vi "Grenzen und Einheit finden.vi"(11 "Ref Auswahlfelder":refnum<vi>[](array[refnum])) -> (0 "Einheit Anzeige":T3, 2 "Grenzen Max":T1 {"Zahlen-Eingabefeld 16" format="%#_5g"; "Zahlen-Eingabefeld 15" format="%#_5g"; "Zahlen-Eingabefeld 14" format="%#_5g"; "Zahlen-Eingabefeld 13" format="%#_5g"; "Zahlen-Eingabefeld 12" format="%#_5g"; "Zahlen-Eingabefeld 11" format="%#_5g"; "Zahlen-Eingabefeld 10" format="%#_5g"; "Zahlen-Eingabefeld 9" format="%#_5g"; "Zahlen-Eingabefeld 8" format="%#_5g"; "Zahlen-Eingabefeld 7" format="%#_5g"; "Zahlen-Eingabefeld 6" format="%#_5g"; "Zahlen-Eingabefeld 5" format="%#_5g"; "Zahlen-Eingabefeld 4" format="%#_5g"; "Zahlen-Eingabefeld 3" format="%#_5g"; "Zahlen-Eingabefeld 2" format="%#_5g"; "Zahlen-Eingabefeld" format="%#_5g"}, 3 "Grenzen Min":T1 {"Zahlen-Eingabefeld 16" format="%#_5g"; "Zahlen-Eingabefeld 15" format="%#_5g"; "Zahlen-Eingabefeld 14" format="%#_5g"; "Zahlen-Eingabefeld 13" format="%#_5g"; "Zahlen-Eingabefeld 12" format="%#_5g"; "Zahlen-Eingabefeld 11" format="%#_5g"; "Zahlen-Eingabefeld 10" format="%#_5g"; "Zahlen-Eingabefeld 9" format="%#_5g"; "Zahlen-Eingabefeld 8" format="%#_5g"; "Zahlen-Eingabefeld 7" format="%#_5g"; "Zahlen-Eingabefeld 6" format="%#_5g"; "Zahlen-Eingabefeld 5" format="%#_5g"; "Zahlen-Eingabefeld 4" format="%#_5g"; "Zahlen-Eingabefeld 3" format="%#_5g"; "Zahlen-Eingabefeld 2" format="%#_5g"; "Zahlen-Eingabefeld" format="%#_5g"})   [LabVIEW 2020, in "Gaszuordnung AO.lvlib"]
uses:
  Gaszuordnung AO.lvlib
  Einheit Anzeige.ctl
  Visualisierungs Elemente/String - Ausgabefeld.ctl
  Grenzen Anzeige.ctl
  Visualisierungs Elemente/Zahlen-Eingabefeld.ctl
  FGV Gaszuordnung Grenzen&Einheit Aktion.ctl
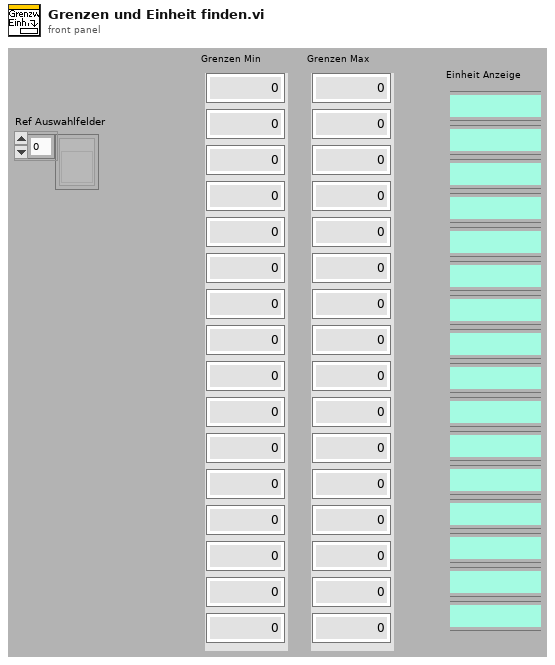
[diagram p1: front panel]
types:
  T1 = typedef "Gaszuordnung AO.lvlib/Grenzen Anzeige.ctl" = cluster{"Zahlen-Eingabefeld":T2, "Zahlen-Eingabefeld 2":T2, "Zahlen-Eingabefeld 3":T2, "Zahlen-Eingabefeld 4":T2, "Zahlen-Eingabefeld 5":T2, "Zahlen-Eingabefeld 6":T2, "Zahlen-Eingabefeld 7":T2, "Zahlen-Eingabefeld 8":T2, "Zahlen-Eingabefeld 9":T2, "Zahlen-Eingabefeld 10":T2, "Zahlen-Eingabefeld 11":T2, "Zahlen-Eingabefeld 12":T2, "Zahlen-Eingabefeld 13":T2, "Zahlen-Eingabefeld 14":T2, "Zahlen-Eingabefeld 15":T2, "Zahlen-Eingabefeld 16":T2}
  T2 = typedef "Zahlen-Eingabefeld.ctl" = sgl
  T3 = typedef "Gaszuordnung AO.lvlib/Einheit Anzeige.ctl" = cluster{"String - Ausgabefeld":T4, "String - Ausgabefeld 2":T4, "String - Ausgabefeld 3":T4, "String - Ausgabefeld 4":T4, "String - Ausgabefeld 5":T4, "String - Ausgabefeld 6":T4, "String - Ausgabefeld 7":T4, "String - Ausgabefeld 8":T4, "String - Ausgabefeld 9":T4, "String - Ausgabefeld 10":T4, "String - Ausgabefeld 11":T4, "String - Ausgabefeld 12":T4, "String - Ausgabefeld 13":T4, "String - Ausgabefeld 14":T4, "String - Ausgabefeld 15":T4, "String - Ausgabefeld 16":T4}
  T4 = typedef "String - Ausgabefeld.ctl" = string
  T5 = typedef "Gaszuordnung AO.lvlib/FGV Gaszuordnung Grenzen&Einheit Aktion.ctl" = enum16{"Lesen", "Schreiben Min", "Schreiben Max", "Laden", "Speichern"}
  T6 = cluster{"[0]":dbl, "[1]":dbl, "[2]":dbl, "[3]":dbl, "[4]":dbl, "[5]":dbl, "[6]":dbl, "[7]":dbl, "[8]":dbl, "[9]":dbl, "[10]":dbl, "[11]":dbl, "[12]":dbl, "[13]":dbl, "[14]":dbl, "[15]":dbl}
  T7 = cluster{"[0]":string, "[1]":string, "[2]":string, "[3]":string, "[4]":string, "[5]":string, "[6]":string, "[7]":string, "[8]":string, "[9]":string, "[10]":string, "[11]":string, "[12]":string, "[13]":string, "[14]":string, "[15]":string}
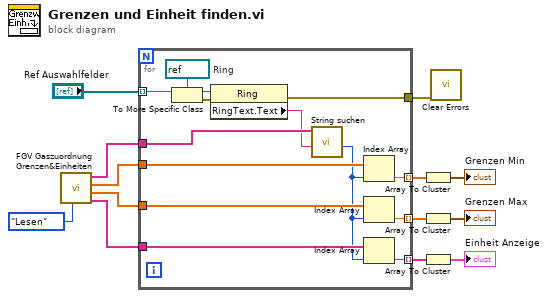
[diagram p0: block diagram]
diagram:
  n1 = call "FGV Gaszuordnung Grenzen&Einheiten.vi"("Aktion"=FGV_Gaszuordnung_Grenzen&Einheit_Aktion."Lesen") -> ("Einheit neu"=w3:string[], "Max neu"=w4:dbl[], "Min neu"=w5:dbl[], "Namen neu"=w6:string[])  [unwired: 2 in, 5 out]
  n2 = for {
    tunnel: "Ref Auswahlfelder" -> [w26] mode=indexing
    tunnel: w6 -> [w18]
    tunnel: w5 -> [w24]
    tunnel: w4 -> [w23]
    tunnel: w3 -> [w22]
    tunnel: [w21] -> w12 mode=indexing
    tunnel: [w20] -> w11 mode=indexing
    tunnel: [w19] -> w10 mode=indexing
    tunnel: [w14] -> w1
    w27 = refnum<vi> refnum  # Ring
    n3 = To More Specific Class(target class=w27, reference=w26) -> (specific class reference=w25:refnum<vi>, error out=w15:errorcluster)  [unwired: 1 in]
    n4 = property class="Ring"(reference=w25, error in=w15) -> (error out=w14:errorcluster, "RingText.Text"=w17:string)  [unwired: 1 out]
    n5 = call "String suchen.vi"("Gasname"=w17, "Such-Namen"=w18) -> ("Index"=w16:i32)  [unwired: 8 in, 1 out]
    n6 = Index Array(array=w24, index=w16) -> (element=w21:dbl)
    n7 = Index Array(array=w23, index=w16) -> (element=w20:dbl)
    n8 = Index Array(array=w22, index=w16) -> (element=w19:string)
  }
  n9 = Array To Cluster(array=w12) -> (cluster=→"Grenzen Min":T6)
  n10 = Array To Cluster(array=w11) -> (cluster=→"Grenzen Max":T6)
  n11 = Array To Cluster(array=w10) -> (cluster=→"Einheit Anzeige":T7)
  n12 = call <vilib>:"Clear Errors.vi"("error in (no error)"=w1) -> ()  [unwired: 5 in, 2 out]
